vi "setHealthAndStatus.vi"(10 "HealthAndStatus":refnum<class "RTHealthAndStatus.lvclass">, 11 "Model in":refnum<class "Model.lvclass">) -> (3 "Model out":refnum<class "Model.lvclass">)   [LabVIEW 2016, in "Model.lvclass"]
uses:
  Model.lvclass
  Common_RT_HealthAndStatus/RTHealthAndStatus/RTHealthAndStatus.lvclass
  Model.lvclass/Model.ctl
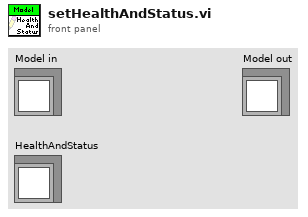
[diagram p1: front panel]
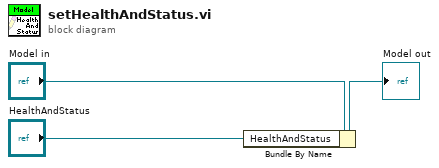
[diagram p0: block diagram]
diagram:
  n1 = Bundle By Name(cluster="Model in", "HealthAndStatus"="HealthAndStatus") -> (→"Model out":refnum<class "Model.lvclass">)
